vi "Tree Map to Tree Control Items RecursiveChild.vi"(7 "Delimiter":string, 9 "Export Options":T1, 10 "Tree Path (Parent, Child)":string[](array[string]), 11 "Tree Map In":T5) -> (0 "error out":errorcluster, 3 "Tree Control Item":T9(array[cluster]))   [LabVIEW 2020, in "Blue Tree Map OpenSource.lvlib"]
uses:
  Blue Tree Map OpenSource.lvlib
  Typedefs/Tree Map.ctl
  Typedefs/Tree Map Data.ctl
  Typedefs/Tree Node Data.ctl
  Typedefs/Attribute Map.ctl
  Typedefs/Tree Map Export Options.ctl
  Typedefs/Tree Map Export Sorting.ctl
  Typedefs/Sort Type.ctl
  Typedefs/Sort AscDesc.ctl
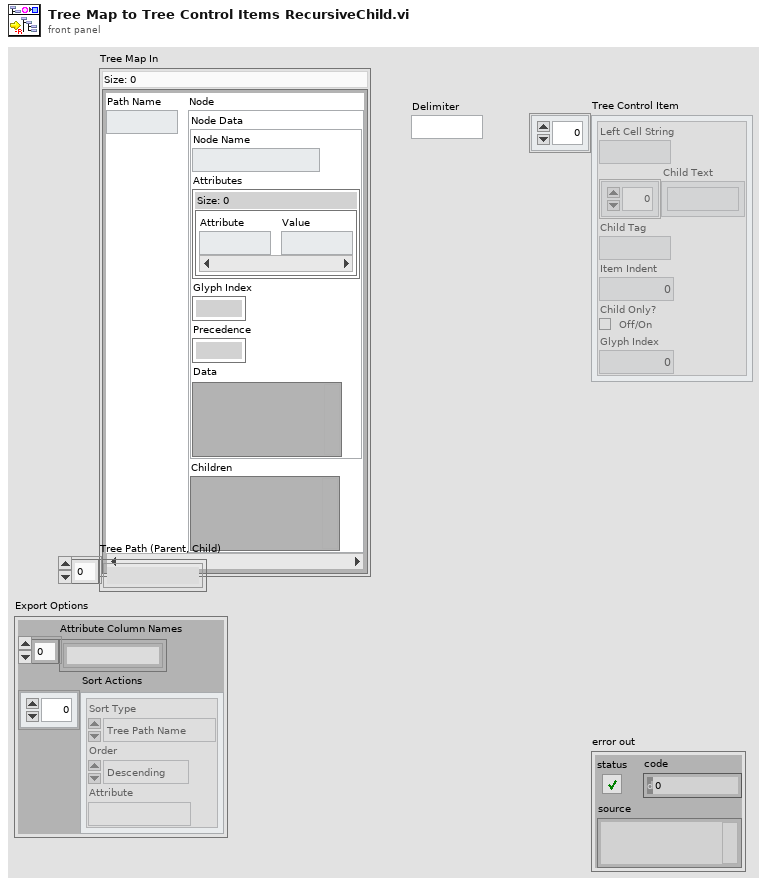
[diagram p1: front panel]
types:
  T1 = typedef "Blue Tree Map OpenSource.lvlib/Tree Map Export Options.ctl" = cluster{"Attribute Column Names":string[], "Sort Actions":T2[]}
  T2 = typedef "Blue Tree Map OpenSource.lvlib/Tree Map Export Sorting.ctl" = cluster{"Sort Type":T3, "Order":T4, "Attribute":string}
  T3 = typedef "Blue Tree Map OpenSource.lvlib/Sort Type.ctl" = enum16{"Tree Path Name", "Node Name", "Attribute", "Precedence"}
  T4 = typedef "Blue Tree Map OpenSource.lvlib/Sort AscDesc.ctl" = enum16{"Descending", "Ascending"}
  T5 = typedef "Blue Tree Map OpenSource.lvlib/Tree Map.ctl" = map{string, T6}
  T6 = typedef "Blue Tree Map OpenSource.lvlib/Tree Map Data.ctl" = cluster{"Node Data":T7, "Children":variant}
  T7 = typedef "Blue Tree Map OpenSource.lvlib/Tree Node Data.ctl" = cluster{"Node Name":string, "Attributes":T8, "Glyph Index":i32, "Precedence":i32, "Data":variant}
  T8 = typedef "Blue Tree Map OpenSource.lvlib/Attribute Map.ctl" = map{string, string}
  T9 = cluster{"Left Cell String":string, "Child Text":string[], "Child Tag":string, "Item Indent":i32, "Child Only?":bool, "Glyph Index":i32}[]
  T10 = cluster{"Left Cell String":string, "Child Text":string[], "Child Tag":string, "Item Indent":i32, "Child Only?":bool, "Glyph Index":i32}
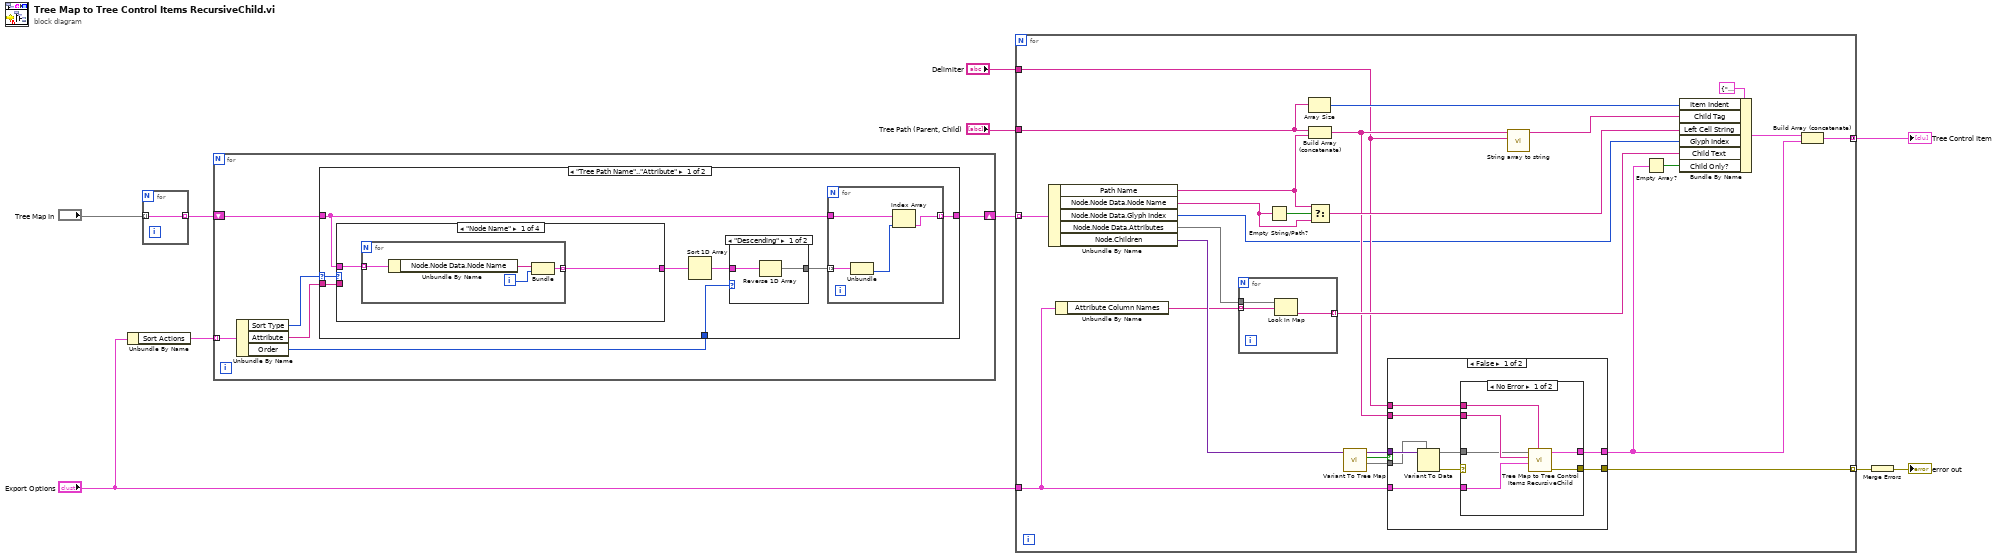
[diagram p0: block diagram]
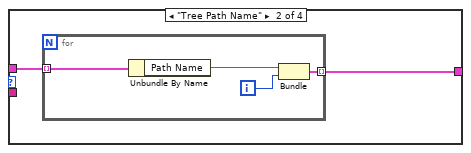
[diagram p2: hidden frame]
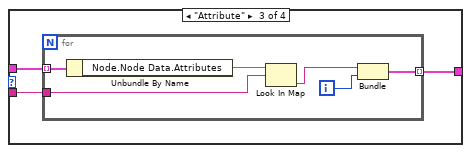
[diagram p3: hidden frame]
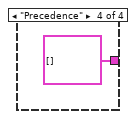
[diagram p4: hidden frame]
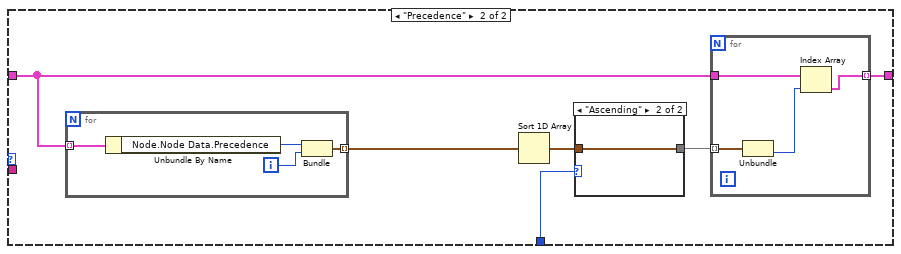
[diagram p6: hidden frame]
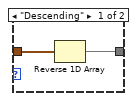
[diagram p7: hidden frame]
diagram:
  n1 = Unbundle By Name("Export Options") -> ("Sort Actions"=w4:T2[])
  n2 = for {
    tunnel: [w11] -> w2 mode=indexing
    tunnel: "Tree Map In" -> [w11] mode=indexing
  }
  n3 = for {
    tunnel: w4 -> [w17] mode=indexing
    shift-right: [w14] -> w1
    shift-left: w2 -> [w15]
    n4 = Unbundle By Name(w17) -> ("Sort Type"=w16:T3, "Attribute"=w12:string, "Order"=w13:T4)
    n5 = case shown="\"Tree Path Name\"..\"Attribute\"" w16 {
      selector: w16 -> [w24 _]
      tunnel: w15 -> [w23 w59]
      tunnel: [w22 w58] -> w14
      tunnel: w13 -> [w21 w57]
      tunnel: w12 -> [w18 _]
      frame "Tree Path Name".."Attribute" {
        n6 = case shown="\"Node Name\"" w24 {
          tunnel: w23 -> [w27 w33 w40 _]
          tunnel: [w26 w32 w39 cluster{"Value":string, i32}[] []] -> w25
          tunnel: w18 -> [_ _ w38 _]
          frame "Node Name" {
            n7 = for {
              tunnel: w27 -> [w31] mode=indexing
              tunnel: [w28] -> w26 mode=indexing
              i -> [w29]
              n8 = Unbundle By Name(w31) -> ("Node.Node Data.Node Name"=w30:string)
              n9 = Bundle("Node Name"=w30, w29) -> (w28:cluster{"Node Name":string, i32})  [unwired: 1 in]
            }
          }
          frame "Tree Path Name" {
            n10 = for {
              tunnel: w33 -> [w37] mode=indexing
              tunnel: [w34] -> w32 mode=indexing
              i -> [w35]
              n11 = Unbundle By Name(w37) -> ("Path Name"=w36:string)
              n12 = Bundle("Path Name"=w36, w35) -> (w34:cluster{"Path Name":string, i32})  [unwired: 1 in]
            }
          }
          frame "Attribute" {
            n13 = for {
              tunnel: w40 -> [w46] mode=indexing
              tunnel: [w44] -> w39 mode=indexing
              tunnel: w38 -> [w42]
              i -> [w45]
              n14 = Unbundle By Name(w46) -> ("Node.Node Data.Attributes"=w43:T8)
              n15 = Look In Map(map=w43, key=w42) -> (value=w41:string)  [unwired: 1 in, 1 out]
              n16 = Bundle("Value"=w41, w45) -> (w44:cluster{"Value":string, i32})  [unwired: 1 in]
            }
          }
          frame "Precedence" {
          }
        }
        n17 = Sort 1D Array(array=w25) -> (sorted array=w20:cluster{"Value":string, i32}[])
        n18 = case shown="\"Descending\"" w21 {
          tunnel: w20 -> [w49 w50]
          tunnel: [w48 w50] -> w19
          frame "Descending" {
            n19 = Reverse 1D Array(array=w49) -> (reversed array=w48:cluster{"Value":string, i32}[])
          }
          frame "Ascending" {
          }
        }
        n20 = for {
          tunnel: w19 -> [w54] mode=indexing
          tunnel: w23 -> [w53]
          tunnel: [w51] -> w22 mode=indexing
          n21 = Unbundle(w54) -> (w52:i32)  [unwired: 1 out]
          n22 = Index Array(array=w53, index=w52) -> (element=w51:cluster{"Path Name":string, "Node":T6})
        }
      }
      frame "Precedence" {
        n23 = for {
          tunnel: w59 -> [w64] mode=indexing
          tunnel: [w61] -> w60 mode=indexing
          i -> [w62]
          n24 = Unbundle By Name(w64) -> ("Node.Node Data.Precedence"=w63:i32)
          n25 = Bundle("Precedence"=w63, w62) -> (w61:cluster{"Precedence":i32, i32})  [unwired: 1 in]
        }
        n26 = Sort 1D Array(array=w60) -> (sorted array=w56:cluster{"Precedence":i32, i32}[])
        n27 = case shown="\"Ascending\"" w57 {
          tunnel: w56 -> [w66 w67]
          tunnel: [w65 w67] -> w55
          frame "Descending" {
            n28 = Reverse 1D Array(array=w66) -> (reversed array=w65:cluster{"Precedence":i32, i32}[])
          }
          frame "Ascending" {
          }
        }
        n29 = for {
          tunnel: w55 -> [w71] mode=indexing
          tunnel: w59 -> [w70]
          tunnel: [w68] -> w58 mode=indexing
          n30 = Unbundle(w71) -> (w69:i32)  [unwired: 1 out]
          n31 = Index Array(array=w70, index=w69) -> (element=w68:cluster{"Path Name":string, "Node":T6})
        }
      }
    }
  }
  n32 = for {
    tunnel: w1 -> [w96] mode=indexing
    tunnel: "Tree Path (Parent, Child)" -> [w87]
    tunnel: [w82] -> w9 mode=concatenating
    tunnel: "Delimiter" -> [w79]
    tunnel: [w74] -> w7 mode=indexing
    tunnel: "Export Options" -> [w73]
    n33 = Unbundle By Name(w96) -> ("Path Name"=w92:string, "Node.Node Data.Node Name"=w91:string, "Node.Node Data.Glyph Index"=w78:i32, "Node.Node Data.Attributes"=w89:T8, "Node.Children"=w94:variant)
    n34 = Unbundle By Name(w73) -> ("Attribute Column Names"=w72:string[])
    n35 = for {
      tunnel: w72 -> [w114] mode=indexing
      tunnel: w89 -> [w115]
      tunnel: [w113] -> w88 mode=indexing
      n36 = Look In Map(map=w115, key=w114) -> (value=w113:string)  [unwired: 1 in, 1 out]
    }
    n37 = Empty String/Path?(string/path=w91) -> (empty?=w93:bool)
    n38 = Array Size(array=w87) -> (size(s)=w86:i32)
    n39 = Build Array (concatenate)(w87, w92) -> (w81:string[])
    n40 = Select(t=w92, s=w93, f=w91) -> (s? t:f=w90:string)
    n41 = call "Variant To Tree Map.vi"("Children"=w94) -> ("Tree Map (Empty)"=w75:T5, "Empty?"=w84:bool, "Children"=w85:variant)  [unwired: 8 in]
    n42 = case shown="False" w84 {
      tunnel: w85 -> [w100 _]
      tunnel: w81 -> [w105 _]
      tunnel: w73 -> [w104 _]
      tunnel: [w103 _] -> w76
      tunnel: w79 -> [w102 _]
      tunnel: [w101 _] -> w74
      tunnel: w75 -> [w99 _]
      frame False {
        n43 = Variant To Data(type=w99, Variant=w100) -> (data=w98:T5, error out=w97:errorcluster)  [unwired: 1 in]
        n44 = case shown="No Error" w97 {
          selector: w97 -> [_ w112]
          tunnel: w105 -> [w111 _]
          tunnel: w104 -> [w110 _]
          tunnel: [w109 _] -> w103
          tunnel: w102 -> [w108 _]
          tunnel: [w107 w112] -> w101
          tunnel: w98 -> [w106 _]
          frame No Error {
            n45 = call "Tree Map to Tree Control Items RecursiveChild.vi"("Delimiter"=w108, "Export Options"=w110, "Tree Path (Parent, Child)"=w111, "Tree Map In"=w106) -> ("error out"=w107:errorcluster, "Tree Control Item"=w109:T9)  [unwired: 6 in]
          }
          frame Error {
          }
        }
      }
      frame True {
      }
    }
    n46 = call "String array to string.vi"("delimiter (\\)"=w79, "Array"=w81) -> ("String"=w80:string)  [unwired: 9 in]
    n47 = Empty Array?(array=w76) -> (empty?=w77:bool)
    n48 = Bundle By Name(cluster=T10 {"Left Cell String"="", "Child Text"=[], "Child Tag"="", "Item Indent"=0, "Child Only?"=FALSE, "Glyph Index"=0} ("Item"), "Item Indent"=w86, "Child Tag"=w80, "Left Cell String"=w90, "Glyph Index"=w78, "Child Text"=w88, "Child Only?"=w77) -> (w83:T10)
    n49 = Build Array (concatenate)(w83, w76) -> (w82:T9)
  }
  "Tree Control Item" <- w9
  n50 = Merge Errors(w7) -> (→"error out":errorcluster)
